vi "PH_Sequencer.set Z6 Beamline Settings.vi"(0 "i ref in":refnum<vi>, 1 "Z6 Beamline State":dbl, 2 "linked?":bool, 5 "error in (no error)":errorcluster) -> (14 "i ref out":refnum<vi>, 19 "error out":errorcluster)   [LabVIEW 2014, in "PH_Sequencer.lvlib"]
doc: "This VI gets whether the Z6 Beamline instance is alive or not."
uses:
  PH_Sequencer.lvlib
  PH_Basics/PH_Common/PH_Common.lvlib
  PH_BL-Master/PH_BL-Master.lvlib
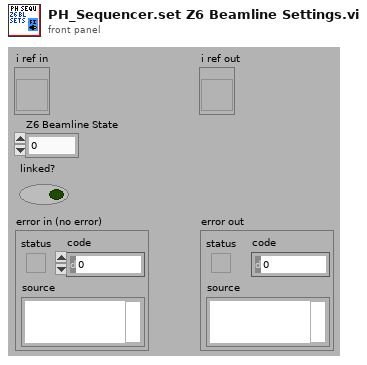
[diagram p1: front panel]
types:
  T1 = typedef "PH_Sequencer.lvlib/PH_Sequencer.i attribute.ctl" = cluster{"GUI Refs":cluster{"Main Off":refnum<vi>, "Fire":refnum<vi>, "Status":refnum<vi>, "Ready":refnum<vi>, "Waiting Time":refnum<vi>, "Timeout":refnum<vi>, "PPMA Ready":refnum<vi>, "Sequencer SM State":refnum<vi>, "PPPA Ready":refnum<vi>, "Calorimeter":refnum<vi>, "Beamline Ready":refnum<vi>, "Clear Beamline":refnum<vi>, "Linkage PPMA Rods":refnum<vi>, "Linkage Current PA":refnum<vi>, "Linkage Current MA":refnum<vi>, "Timing Ready":refnum<vi>, "State Timing":refnum<vi>, "Force Timing":refnum<vi>, "PSDB Shot Comment":refnum<vi>, "State PA Backreflection":refnum<vi>, "Beamline Z6 Ready":refnum<vi>, "Clear Z6 Beamline":refnum<vi>, "Sequence length":refnum<vi>, "Timing Mode":refnum<vi>, "Slow Trigger Settings":refnum<vi>, "Experiment Description":refnum<vi>, "State PSDB":refnum<vi>, "PSDB Ready":refnum<vi>, "Set PSDB Settings":refnum<vi>, "Get PSDB Info":refnum<vi>, "Take Snapshot":refnum<vi>, "Shottype":refnum<vi>, "Experiment":refnum<vi>, "Phase Frontends":refnum<vi>, "PP 45mm PILC in use":refnum<vi>}, "Status Info":cluster{"Machine Status":T2, "WaitingTime":i32, "Timeout":bool}, "Readyness":cluster{"Ready to shot":bool, "PPMA Ready":bool, "PPPA Ready":bool, "BL Ready":bool, "Timing Ready":bool, "BL Z6 Ready":bool, "PSDBReady":bool}, "Instancenames":cluster{"PPMA Rods":string, "PP Current Meas":string, "PH Beamline Chief":string, "PA Backrefl Meas":string, "Z6 Beamline Chief":string}, "Data to read":bool, "Calorimeter":cluster{"Instancename":string, "On":bool, "linked":bool}, "Linkage":cluster{"PPMA Rods":bool, "PP Current Meas":bool, "PHELIX Beamline Chief":bool, "PA Backrefl Meas":bool, "Z6 Beamline Chief":bool}, "Timing":cluster{"Instance":string, "linked":bool, "Status":T2, "Timing Mode":T3, "Slow Trigger Settings":T4, "Info available":cluster{"ext SlowTrigger":bool, "T2":bool, "Mode":bool, "Delay Slow Trigger":bool, "Phase FEs":bool}, "FE Phase":T5}, "Service ID R2S":i32, "PSDB":cluster{"Controller Instance":string, "Controller Status":T2, "Controller linked":bool, "Settings acknowledged":bool, "Current Experiment ID":i16, "Current Shot Type":i16, "Current Comment":string, "Remember Settings":bool, "Write 2 early":bool}, "PSDB Data":cluster{"Main Off?":bool, "Sequence Length":dbl, "Sequence startet":timestamp}, "6P 4Q Positions":cluster{"Instancename":string, "linked":bool, "Position":T6}[], "PUs":T7[]}
  T2 = typedef "PH_StatusHandler.lvlib/PH_StatusHandler.Status.ctl" = i16
  T3 = typedef "PH_Timing.lvlib/PH_Timing.Timing Mode.ctl" = cluster{"T2":i16, "Modeselector":enum32{"10 Hz", "0.5 Hz", "Shot"}}
  T4 = typedef "PH_Timing.lvlib/PH_Timing.Slow Trigger Settings.ctl" = cluster{"Delay":dbl, "externally triggered?":bool}
  T5 = typedef "PH_Timing.lvlib/PH_Timing.Phase FEs.ctl" = cluster{"Phase":dbl}
  T6 = typedef "PH_4_Pos_Selector.lvlib/PH_4_Pos_Selector.Position Selector.ctl" = u16
  T7 = typedef "PH_Sequencer.lvlib/PH_Sequencer.Head.ctl" = cluster{"PowerUnit":T8, "GUI Ref":refnum<vi>, "Information":T9, "linked?":bool, "GUI Ref Current Voltage":refnum<vi>}
  T8 = typedef "PH_PP_Common.lvlib/PH_PP_Common.PUs.ctl" = enum16{"no Info", "PA-19mm-1", "PA-19mm-2", "PA-45mm-PILC", "PA-45mm-MAIN", "MA-PU-1", "MA-PU-2", "MA-PU-3", "MA-PU-4", "MA-PU-5", "MA-PU-6", "MA-FR", "MA-PILC", "PA-45mm-DP"}
  T9 = typedef "PH_Sequencer.lvlib/PH_Sequencer.PU Information.ctl" = cluster{"State":T2, "Waiting Time [s]":dbl, "PU State SM":T10, "PU Timeout SM":T10}
  T10 = typedef "PH_PowerUnit_BaseClass.lvlib/PH_PowerUnit_BaseClass.SM States.ctl" = enum16{".", "Stand by", "Switch PU on", "Configure", "Set Default Voltage", "Set STANDBY", "Set READY", "Wait for Shot Cmd", "Open Dump Rods", "Open Ross Relais", "Close Ross Relais", "Switch PSU on", "Switch PSU off", "Charge", "Switch GD Channel on", "Close Dump Rods", "Rods-TO", "RR-TO", "PSU-TO", "Trigger-TO"}
  T11 = cluster{"Z6 Beamline Chief":bool, "linked?":bool}
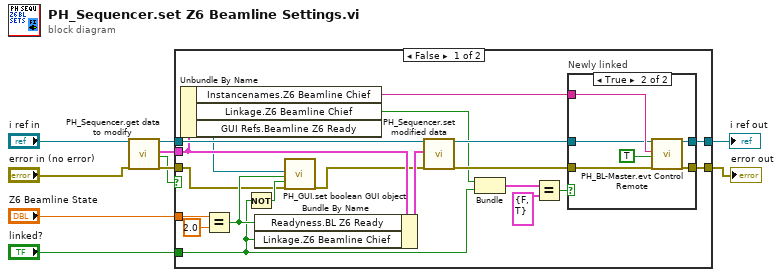
[diagram p0: block diagram]
diagram:
  n1 = call "PH_Sequencer.get data to modify.vi"("i ref in"="i ref in", "error in (no error)"="error in (no error)") -> ("i ref out"=w8:refnum<vi>, "i attribute"=w10:T1, "timed out"=w5:bool, "error out"=w6:errorcluster)  [unwired: 14 in]
  n2 = case shown="False" w5 {
    tunnel: w8 -> [w26 w40]
    tunnel: [w28 w40] -> w3
    tunnel: w6 -> [w19 w39]
    tunnel: [w27 w39] -> w2
    tunnel: w10 -> [w25 _]
    tunnel: "linked?" -> [w12 _]
    tunnel: "Z6 Beamline State" -> [w24 _]
    frame False {
      n3 = Unbundle By Name(w25) -> ("Instancenames.Z6 Beamline Chief"=w17:string, "Linkage.Z6 Beamline Chief"=w11:bool, "GUI Refs.Beamline Z6 Ready"=w22:refnum<vi>)
      n4 = Equal?(x=w24, y=2.0) -> (x = y?=w21:bool)
      n5 = Not(x=w12) -> (.not. x?=w20:bool)
      n6 = Bundle By Name(cluster=w25, "Readyness.BL Z6 Ready"=w21, "Linkage.Z6 Beamline Chief"=w12) -> (w30:T1)
      n7 = call "PH_GUI.set boolean GUI object.vi"("Boolean Knob GUI Ref"=w22, "Value"=w21, "Blinking? (false)"=w20, "error in (no error)"=w19) -> ("error out"=w18:errorcluster)  [unwired: 15 in]
      n8 = call "PH_Sequencer.set modified data.vi"("i ref in"=w26, "i attribute"=w30, "error in (no error)"=w18) -> ("i ref out"=w16:refnum<vi>, "error out"=w29:errorcluster)  [unwired: 15 in]
      n9 = Bundle("Z6 Beamline Chief"=w11, "linked?"=w12) -> (w15:T11)  [unwired: 1 in]
      n10 = Equal?(x=w15, y=cluster{"Beamline":bool, "linked?":bool} {"Beamline"=FALSE, "linked?"=TRUE}) -> (x = y?=w13:bool)
      n11 = case "Newly linked" shown="True" w13 {
        tunnel: w29 -> [w31 w38]
        tunnel: [w32 w37] -> w28
        tunnel: [w31 w36] -> w27
        tunnel: w17 -> [_ w35]
        tunnel: w16 -> [w32 w34]
        frame False {
        }
        frame True {
          n12 = call "PH_BL-Master.evt Control Remote.vi"("i ref in"=w34, "Instance"=w35, "Control Remote"=TRUE, "error in (no error)"=w38) -> ("i ref out"=w37:refnum<vi>, "error out"=w36:errorcluster)  [unwired: 14 in]
        }
      }
    }
    frame True {
    }
  }
  "i ref out" <- w3
  "error out" <- w2
